vi "Read magnetometer.vi"(8 "error in (no error)":errorcluster, 11 "Accelerometer":T1) -> (0 "error out":errorcluster, 2 "read data":u8[](array[numeric]), 3 "Accelerometer out":T1)   [LabVIEW 2013]
doc: "Use this template to build a VI to use as a subVI."
uses:
  AccelerometerSPI.ctl
  <vilib>/ni845x/ni845x.llb/ni845xControl.ctl
  <vilib>/ni845x/ni845x.llb/ni845xSpiConfiguration.ctl
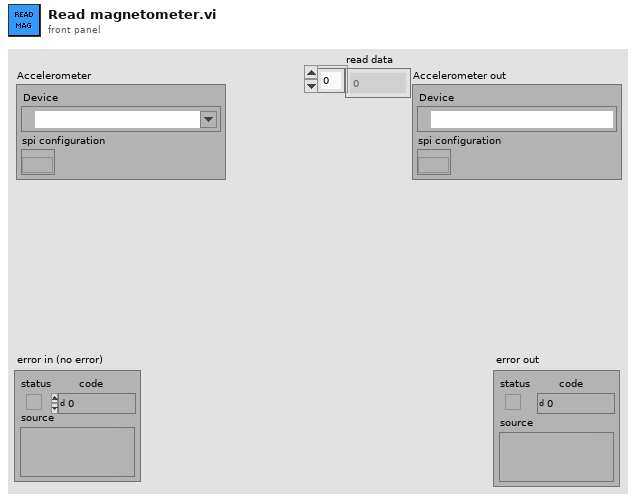
[diagram p1: front panel]
types:
  T1 = typedef "AccelerometerSPI.ctl" = cluster{"Device":T2, "spi configuration":T3}
  T2 = typedef "ni845xControl.ctl" = refnum<k21>
  T3 = typedef "ni845xSpiConfiguration.ctl" = refnum<k20>
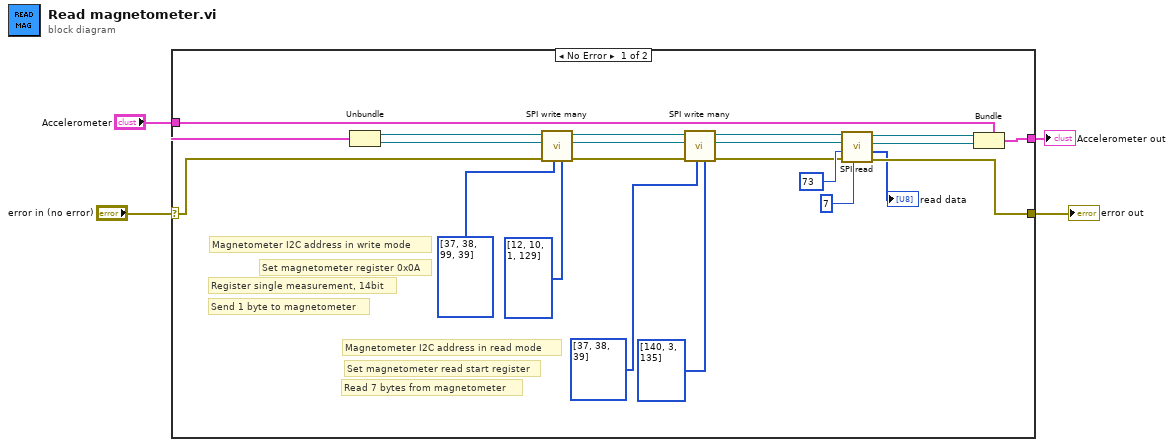
[diagram p0: block diagram]
diagram:
  n1 = case shown="No Error" "error in (no error)" {
    selector: "error in (no error)" -> [w11 w27]
    tunnel: [w21 w27] -> w3
    tunnel: "Accelerometer" -> [w24 w26]
    tunnel: [w25 w26] -> w1
    frame No Error {
      # "Read 7 bytes from magnetometer"
      # "Set magnetometer read start register"
      # "Magnetometer I2C address in read mode"
      # "Send 1 byte to magnetometer"
      # "Register single measurement, 14bit"
      # "Set magnetometer register 0x0A"
      # "Magnetometer I2C address in write mode"
      n2 = Unbundle(w24) -> ("Device"=w13:T2, "spi configuration"=w12:T3)
      n3 = call "SPI write many.vi"("values"=u8[] [12, 10, 1, 129] ("addresses"), "addresses"=u8[] [37, 38, 99, 39], "error in (no error)"=w11, "spi configuration in"=w12, "Device ref in"=w13) -> ("error out"=w10:errorcluster, "spi configuration out"=w9:T3, "Device ref out"=w8:T2)  [unwired: 4 in]
      n4 = call "SPI write many.vi"("values"=u8[] [140, 3, 135] ("addresses"), "addresses"=u8[] [37, 38, 39], "error in (no error)"=w10, "spi configuration in"=w9, "Device ref in"=w8) -> ("error out"=w5:errorcluster, "spi configuration out"=w6:T3, "Device ref out"=w7:T2)  [unwired: 4 in]
      n5 = call "SPI read.vi"("Number of bytes"=7, "error in (no error)"=w5, "Address"=73, "spi configuration in"=w6, "Device ref in"=w7) -> ("error out"=w21:errorcluster, "read data"=→"read data":u8[], "spi configuration out"=w22:T3, "Device ref out"=w23:T2)  [unwired: 3 in]
      n6 = Bundle(cluster=w24, "Device"=w23, "spi configuration"=w22) -> (w25:T1)
    }
    frame Error {
    }
  }
  "error out" <- w3
  "Accelerometer out" <- w1
